vi "PXISlot Test.vi"() -> ()   [LabVIEW 2015]
uses:
  Type Defs/General PXISlot XControl/PXISlotGP.xctl
  Type Defs/PXISlot XControl/Connector Type.ctl
panel:
  in  "change":bool
  in  "rename":bool
  in  "show unused":bool
  in  "PXISlotGP":cluster{"Outputs":string[], "Inputs":string[]}(xcontrol)
  in  "stop":bool
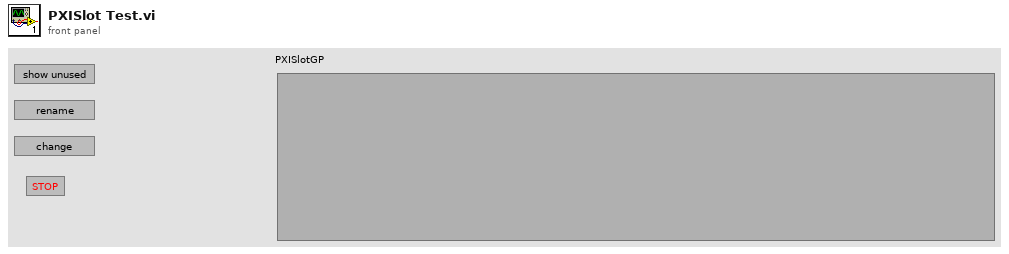
[diagram p1: front panel]
types:
  T1 = typedef "Connector Type.ctl" = enum16{"None", "PXI-4461", "BNC-2110", "BNC-2090"}
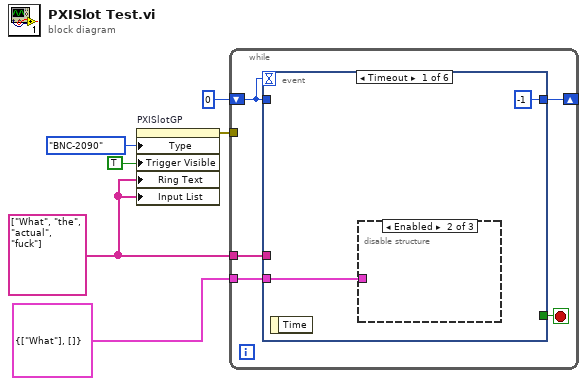
[diagram p0: block diagram]
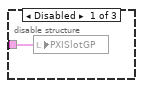
[diagram p2: hidden frame]
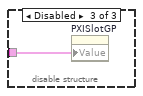
[diagram p3: hidden frame]
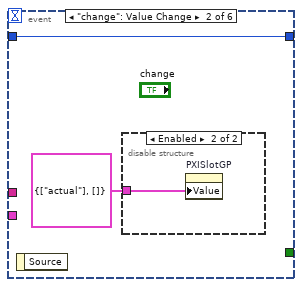
[diagram p4: hidden frame]
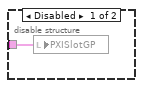
[diagram p5: hidden frame]
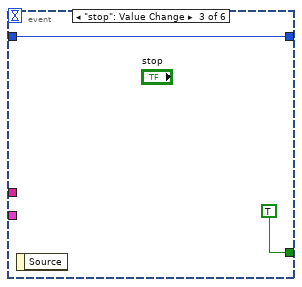
[diagram p6: hidden frame]
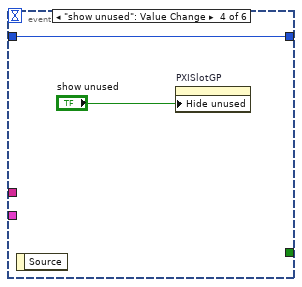
[diagram p7: hidden frame]
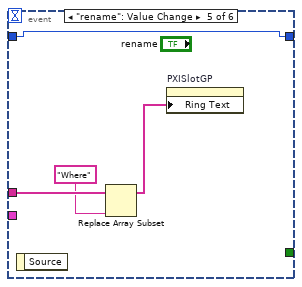
[diagram p8: hidden frame]
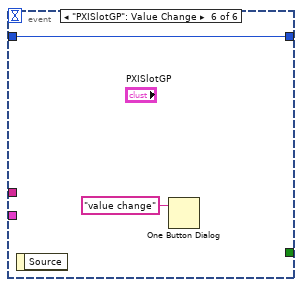
[diagram p9: hidden frame]
diagram:
  w3 = string[] ["What", "the", "actual", "fuck"] ("Output Items")
  n1 = property on="PXISlotGP" class="PXISlotGP (strict)"("Type"=Connector_Type."BNC-2090", "Trigger Visible"=TRUE, "Ring Text"=w3, "Input List"=w3) -> (error out=w4:errorcluster)  [unwired: 2 in, 1 out]
  n2 = while {
    tunnel: w4 -> [_]
    tunnel: w3 -> [w10]
    shift-right: [w8] -> _
    shift-left: 0 -> [w9]
    tunnel: cluster{"Outputs":string[], "Inputs":string[]} {"Outputs"=["What"], "Inputs"=[]} ("PXISlotGP") -> [w7]
    stop <- w11 stop-if-true
    n3 = event shown="[0] Timeout" {
      selector: _ -> [_ _ _ _ _ _]
      dyn-events: _ -> [_ _ _ _ _ _]
      timeout: w9 -> [_ _ _ _ _ _]
      tunnel: [_ _ TRUE _ _ _] -> w11
      tunnel: w10 -> [_ _ _ _ w27 _]
      tunnel: w9 -> [_ w17 w20 w22 w24 w28]
      tunnel: [-1 w17 w20 w22 w24 w28] -> w8
      tunnel: w7 -> [w12 _ _ _ _ _]
      event Timeout {
        n4 = event-data() -> ()  [unwired: 1 in, 1 out]
        n5 = disable-structure shown="Enabled" {
          disable-tunnel: w12 -> [w14 _ w15]
          frame Disabled {
            n6 = local write "PXISlotGP"(w14) -> ()
          }
          frame Enabled {
          }
          frame Disabled {
            n7 = property on="PXISlotGP" class="PXISlotGP (strict)"("Value"=w15) -> ()  [unwired: 2 in, 2 out]
          }
        }
      }
      event "change": Value Change {
        n8 = event-data() -> ()  [unwired: 1 in, 1 out]
        n9 = disable-structure shown="Enabled" {
          disable-tunnel: cluster{"Outputs":string[], "Inputs":string[]} {"Outputs"=["actual"], "Inputs"=[]} ("PXISlotGP") -> [w18 w19]
          frame Disabled {
            n10 = local write "PXISlotGP"(w18) -> ()
          }
          frame Enabled {
            n11 = property on="PXISlotGP" class="PXISlotGP (strict)"("Value"=w19) -> ()  [unwired: 2 in, 2 out]
          }
        }
      }
      event "stop": Value Change {
        n12 = event-data() -> ()  [unwired: 1 in, 1 out]
      }
      event "show unused": Value Change {
        n13 = event-data() -> ()  [unwired: 1 in, 1 out]
        n14 = property on="PXISlotGP" class="PXISlotGP (strict)"("Hide unused"="show unused") -> ()  [unwired: 2 in, 2 out]
      }
      event "rename": Value Change {
        n15 = event-data() -> ()  [unwired: 1 in, 1 out]
        n16 = Replace Array Subset(array=w27, new element="Where" ("new element/subarray")) -> (w25:string[])  [unwired: 1 in]
        n17 = property on="PXISlotGP" class="PXISlotGP (strict)"("Ring Text"=w25) -> ()  [unwired: 2 in, 2 out]
      }
      event "PXISlotGP": Value Change {
        n18 = event-data() -> ()  [unwired: 1 in, 1 out]
        n19 = One Button Dialog(message="value change") -> ()  [unwired: 1 in, 1 out]
      }
    }
  }
